vi "Send and Receive.vi"(6 "timeout (ms) [500]":i32, 8 "error in (no error)":errorcluster, 9 "params":variant, 10 "Command in":string, 11 "Instrument in":refnum<class "Instrument.lvclass">) -> (0 "error out":errorcluster, 1 "Data out":variant, 2 "Command out":string, 3 "Instrument out":refnum<class "Instrument.lvclass">)   [LabVIEW 2019, in "Instrument.lvclass"]
uses:
  Instrument.lvclass
  Instrument.lvclass/Instrument.ctl
  <userlib>/LevyLab/RemoteControl/RemoteControl.lvclass
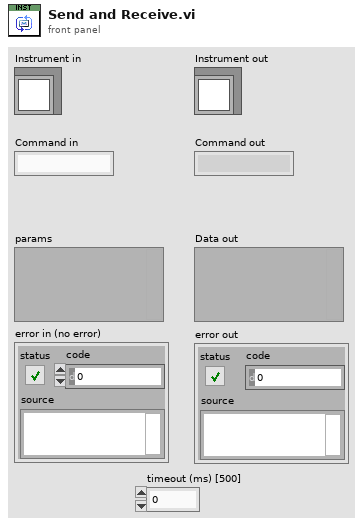
[diagram p1: front panel]
types:
  T1 = typedef "Instrument.lvclass/Dependencies--Cluster.ctl" = cluster{"RemoteControl":refnum<class "RemoteControl.lvclass">, "Logger.Error":refnum<class "Logger.Error.lvclass">, "Logger.PGSQL":refnum<class "Logger.PGSQL.lvclass">, "Configuration":refnum<class "Configuration.lvclass">}
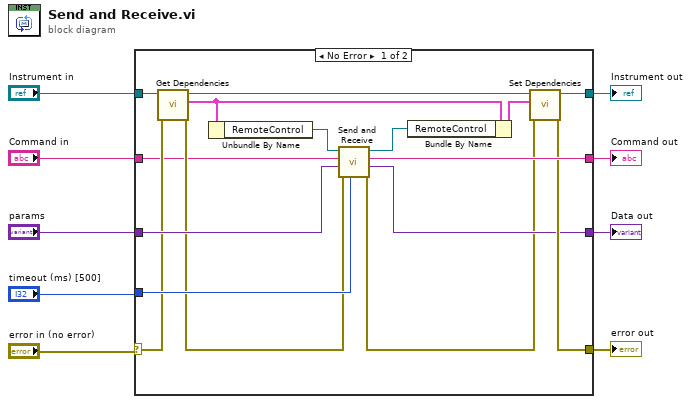
[diagram p0: block diagram]
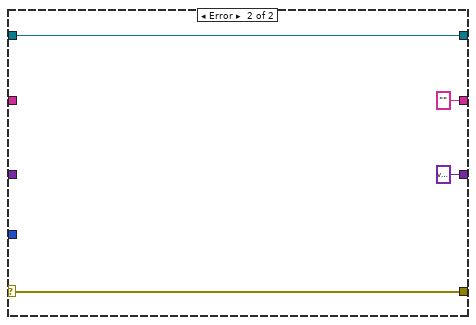
[diagram p2: hidden frame]
diagram:
  n1 = case shown="No Error" "error in (no error)" {
    selector: "error in (no error)" -> [w18 w29]
    tunnel: "Instrument in" -> [w22 w28]
    tunnel: "timeout (ms) [500]" -> [w25 _]
    tunnel: "params" -> [w24 _]
    tunnel: "Command in" -> [w10 _]
    tunnel: [w19 w28] -> w5
    tunnel: [w17 w29] -> w4
    tunnel: [w23 "" ("Command out")] -> w3
    tunnel: [w14 variant ("Data out")] -> w2
    frame No Error {
      n2 = call "Get Dependencies.vi"("error in (no error)"=w18, "Instrument in"=w22) -> ("error out"=w15:errorcluster, "Dependencies"=w16:T1, "Instrument out"=w20:refnum<class "Instrument.lvclass">)  [unwired: 7 in]
      n3 = Unbundle By Name(w16) -> ("RemoteControl"=w12:refnum<class "RemoteControl.lvclass">)
      n4 = call <userlib>:"Send and Receive.vi"("timeout (ms) [500]"=w25, "error in (no error)"=w15, "Data"=w24, "Command"=w10, "RemoteControl in"=w12) -> ("error out"=w13:errorcluster, "Data out"=w14:variant, "Command out"=w23:string, "RemoteControl out"=w11:refnum<class "RemoteControl.lvclass">)  [unwired: 3 in]
      n5 = Bundle By Name(cluster=w16, "RemoteControl"=w11) -> (w21:T1)
      n6 = call "Set Dependencies.vi"("error in (no error)"=w13, "Dependencies"=w21, "Instrument in"=w20) -> ("error out"=w17:errorcluster, "Instrument out"=w19:refnum<class "Instrument.lvclass">)  [unwired: 7 in]
    }
    frame Error {
    }
  }
  "Data out" <- w2
  "error out" <- w4
  "Command out" <- w3
  "Instrument out" <- w5
